vi "TCP-IP Mgr.Get Config.vi"(8 "error in":errorcluster, 10 "Default Config":T1={"IP"="127.0.0.1", "Port"=8500, "Listener"=FALSE, "Enable"=FALSE}, 11 "Path":path=path "C:/TestExec/Config/TESocket.ini") -> (0 "error out":errorcluster, 2 "Config Out":T1={"IP"="127.0.0.1", "Port"=8500, "Listener"=FALSE, "Enable"=FALSE})   [LabVIEW 2024, in "EQMF.lvlib" / "TCP-IP.lvlib"]
uses:
  TCP-IP.lvlib
  TCP-IP Mgr.Config.ctl
  <vilib>/Utility/config.llb/Read Key (String).vi
  <vilib>/Utility/config.llb/Write Key (String).vi
  <vilib>/Utility/config.llb/Read Key (I32).vi
  <vilib>/Utility/config.llb/Write Key (I32).vi
  <vilib>/Utility/config.llb/Read Key (Boolean).vi
  <vilib>/Utility/config.llb/NI_LVConfig.lvlib
  Files/File Utils.lvlib
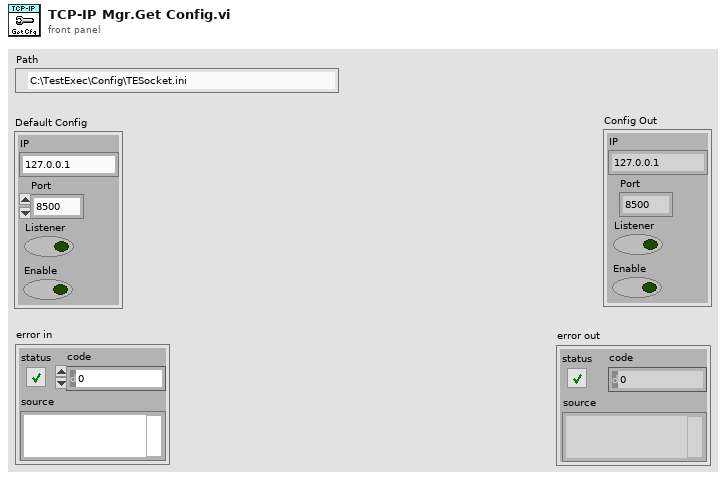
[diagram p1: front panel]
types:
  T1 = typedef "EQMF.lvlib/TCP-IP.lvlib/TCP-IP Mgr.Config.ctl" = cluster{"IP":string, "Port":u16, "Listener":bool, "Enable":bool}
  T2 = typedef "NI_LVConfig.lvlib/Config Data RefNum.ctl" = refnum<k1>
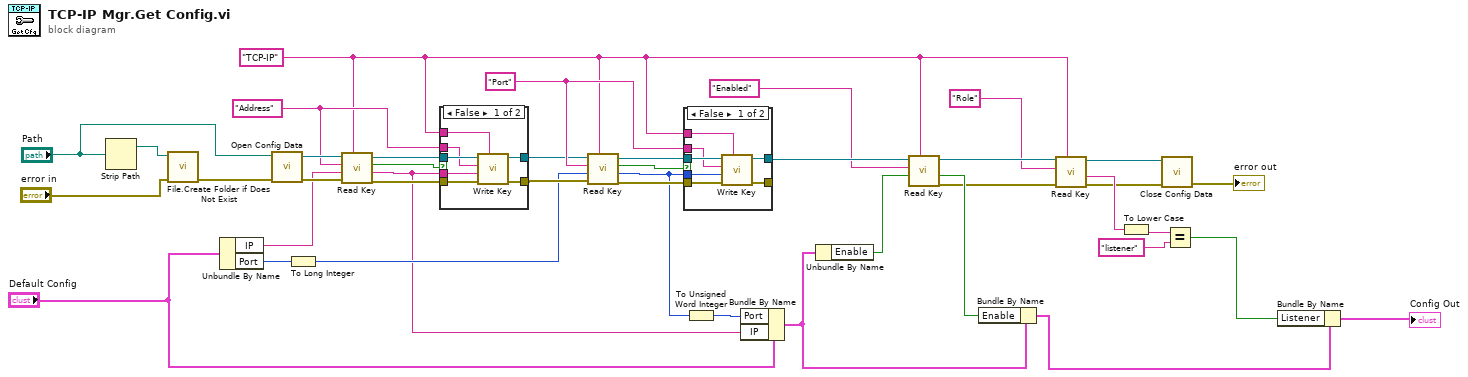
[diagram p0: block diagram]
diagram:
  w30 = "Port"
  w35 = "Address"
  w10 = "TCP-IP"
  n1 = Strip Path(path="Path") -> (stripped path=w22:path)  [unwired: 1 out]
  n2 = call "File.Create Folder if Does Not Exist.vi"("error in"="error in", "Path"=w22) -> ("error out"=w20:errorcluster)  [unwired: 7 in, 2 out]
  n3 = Unbundle By Name("Default Config") -> ("IP"=w39:string, "Port"=w38:u16)
  n4 = call <vilib>:"Open Config Data.vi"("error in (no error)"=w20, "configuration file path"="Path") -> ("error out"=w41:errorcluster, "refnum"=w40:T2)  [unwired: 7 in, 1 out]
  n5 = To Long Integer(number=w38) -> (32bit integer=w26:i32)
  n6 = call-poly <vilib>:"Read Key.vi"("section"=w10, "error in (no error)"=w41, "default value"=w39, "key"=w35, "refnum"=w40) -> ("error out"=w36:errorcluster, "value"=w24:string, "found?"=w33:bool, "refnum out"=w34:T2)  [unwired: 3 in]
  n7 = case shown="False" w33 {
    tunnel: w36 -> [w48 w49]
    tunnel: w24 -> [w47 _]
    tunnel: w35 -> [w45 _]
    tunnel: w34 -> [w46 w50]
    tunnel: w10 -> [w44 _]
    tunnel: [w43 w50] -> w28
    tunnel: [w42 w49] -> w27
    frame False {
      n8 = call-poly <vilib>:"Write Key.vi"("section"=w44, "error in (no error)"=w48, "value"=w47, "key"=w45, "refnum"=w46) -> ("error out"=w42:errorcluster, "refnum out"=w43:T2)  [unwired: 4 in, 1 out]
    }
    frame True {
    }
  }
  n9 = call-poly <vilib>:"Read Key.vi"("section"=w10, "error in (no error)"=w27, "default value"=w26, "key"=w30, "refnum"=w28) -> ("error out"=w29:errorcluster, "value"=w25:i32, "found?"=w32:bool, "refnum out"=w31:T2)  [unwired: 3 in]
  n10 = case shown="False" w32 {
    tunnel: w29 -> [w57 w58]
    tunnel: w25 -> [w56 _]
    tunnel: w30 -> [w54 _]
    tunnel: w31 -> [w55 w59]
    tunnel: w10 -> [w53 _]
    tunnel: [w52 w59] -> w16
    tunnel: [w51 w58] -> _
    frame False {
      n11 = call-poly <vilib>:"Write Key.vi"("section"=w53, "error in (no error)"=w57, "value"=w56, "key"=w54, "refnum"=w55) -> ("error out"=w51:errorcluster, "refnum out"=w52:T2)  [unwired: 4 in, 1 out]
    }
    frame True {
    }
  }
  n12 = To Unsigned Word Integer(number=w25) -> (unsigned 16bit integer=w18:u16)
  n13 = Bundle By Name(cluster="Default Config", "Port"=w18, "IP"=w24) -> (w3:T1)
  n14 = Unbundle By Name(w3) -> ("Enable"=w17:bool)
  n15 = call-poly <vilib>:"Read Key.vi"("section"=w10, "default value"=w17, "key"="Enabled", "refnum"=w16) -> ("error out"=w11:errorcluster, "value"=w14:bool, "refnum out"=w13:T2)  [unwired: 4 in, 1 out]
  n16 = Bundle By Name(cluster=w3, "Enable"=w14) -> (w2:T1)
  n17 = call-poly <vilib>:"Read Key.vi"("section"=w10, "error in (no error)"=w11, "key"="Role", "refnum"=w13) -> ("error out"=w6:errorcluster, "value"=w7:string, "refnum out"=w5:T2)  [unwired: 4 in, 1 out]
  n18 = To Lower Case(string=w7) -> (all lower case string=w8:string)
  n19 = call <vilib>:"Close Config Data.vi"("error in (no error)"=w6, "refnum"=w5) -> ("error out"=→"error out":errorcluster)  [unwired: 8 in, 1 out]
  n20 = Equal?(x=w8, y="listener") -> (x = y?=w4:bool)
  n21 = Bundle By Name(cluster=w2, "Listener"=w4) -> (→"Config Out":T1)
